vi "Position_Test.vi"() -> (3 "Failed?":bool)   [LabVIEW 2017, in "WordManipulationTests.lvlib"]
uses:
  WordManipulationTests.lvlib
  Utilities/WordManipulationLibrary.lvlib
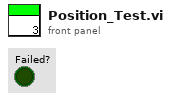
[diagram p1: front panel]
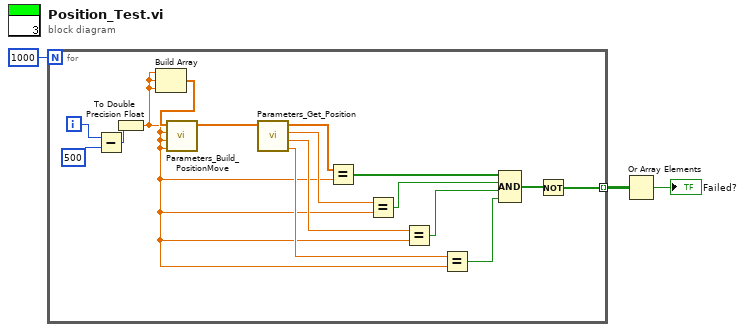
[diagram p0: block diagram]
diagram:
  n1 = for {
    N: 1000 -> [_]
    tunnel: [w9] -> w2 mode=indexing
    i -> [w8]
    n2 = Subtract(x=w8, y=500) -> (x-y=w7:i32)
    n3 = To Double Precision Float(number=w7) -> (double precision float=w4:dbl)
    n4 = Build Array(w4, w4, w4) -> (w5:dbl[])
    n5 = call "Parameters_Build_PositionMove.vi"("Acceleration Jerk"=w4, "Acceleration"=w4, "Velocity"=w4, "Positions"=w5) -> ("Parameters"=w19:dbl[])  [unwired: 7 in]
    n6 = call "Parameters_Get_Position.vi"("Parameters"=w19) -> ("Acceleration Jerk"=w15:dbl, "Acceleration"=w16:dbl, "Velocity"=w17:dbl, "Target Position"=w18:dbl[])  [unwired: 7 in]
    n7 = Equal?(x=w18, y=w4) -> (x = y?=w14:bool[])
    n8 = Equal?(x=w17, y=w4) -> (x = y?=w13:bool)
    n9 = Equal?(x=w16, y=w4) -> (x = y?=w12:bool)
    n10 = Equal?(x=w15, y=w4) -> (x = y?=w11:bool)
    n11 = Compound Arithmetic op=AND(w14, w13, w12, w11) -> (w10:bool[])
    n12 = Not(x=w10) -> (.not. x?=w9:bool[])
  }
  n13 = Or Array Elements(Boolean array=w2) -> (logical OR=→"Failed?":bool)
